vi "PB_VLIW_diagnostics4.vi"(3 "error in \n(no error)":errorcluster, 6 "VLIW Array In":T1(array[cluster]) {"OP Code" format="%.0x"; "Output Bits" format="%.0x"}) -> (0 "error out":errorcluster, 2 "Total Time":dbl=50.0 format="%.2p")   [LabVIEW 2012, in "SubVIs.lvlib"]
doc: "This vi obtains information about a \"VLIW Array\".\n\nIt's inputs are:\n1) the \"VLIW Array\"\n2) error in\nIt's outputs are:\n1) the total time for the sequence\n2) the total number of AO updates for each different AO/DO device specified in the HW Globals array\n3) error out. \n\n\nThe Jump, Return, and GoTo diagnostics are not supported, and attempting to determine diagnostics on an array that contains these commands will generate and error. If there is an error on the input, the diagnostics are not calculated.\n\nThis vi uses the globally defined variables in \"PB_defines\"."
uses:
  PB_defines.vi
  SubVIs.lvlib
  PulseBlaster.lvlib
panel:
  in  "Start loop time":dbl format="%.2p"
  in  "# of loops":u32
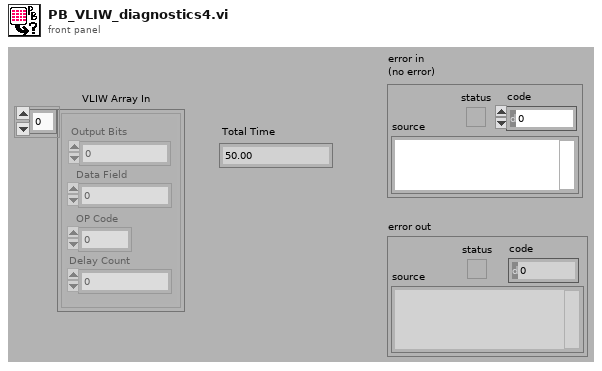
[diagram p1: front panel]
types:
  T1 = cluster{"Output Bits":u32, "Data Field":u32, "OP Code":u8, "Delay Count":u32}[]
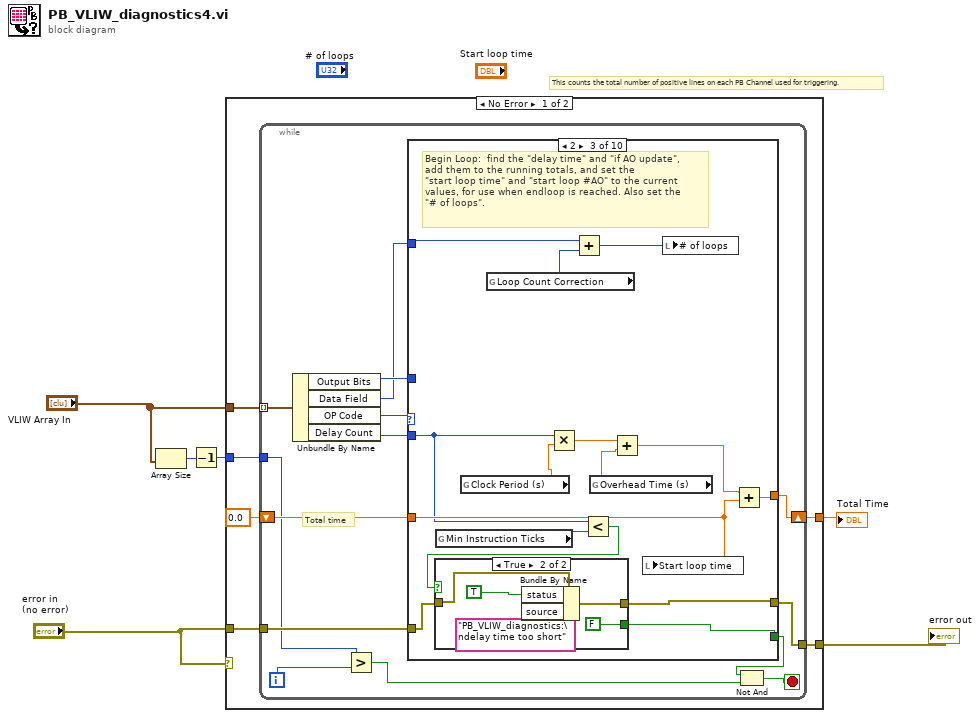
[diagram p0: block diagram]
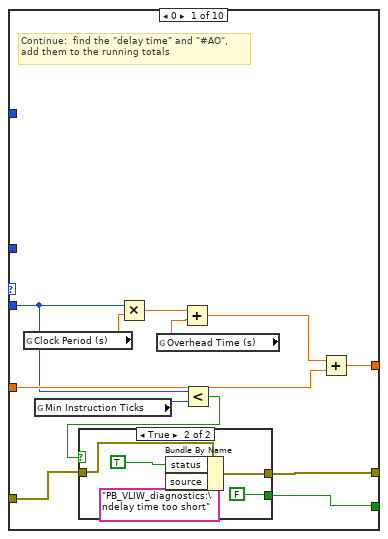
[diagram p2: hidden frame]
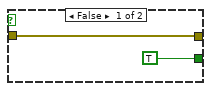
[diagram p3: hidden frame]
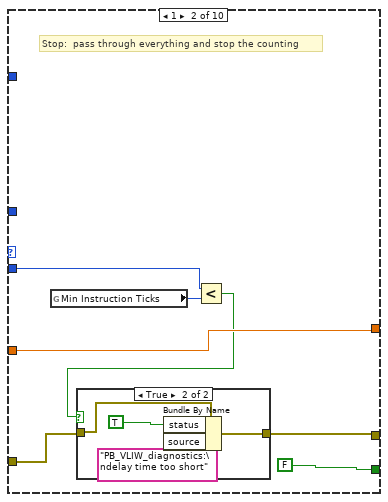
[diagram p4: hidden frame]
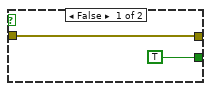
[diagram p6: hidden frame]
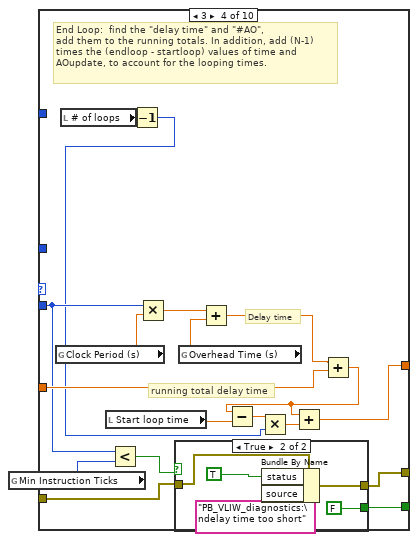
[diagram p7: hidden frame]
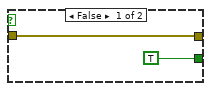
[diagram p8: hidden frame]
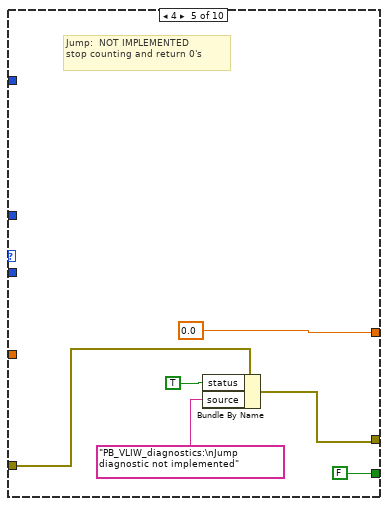
[diagram p9: hidden frame]
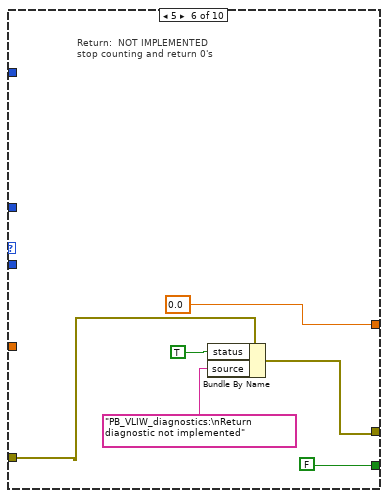
[diagram p10: hidden frame]
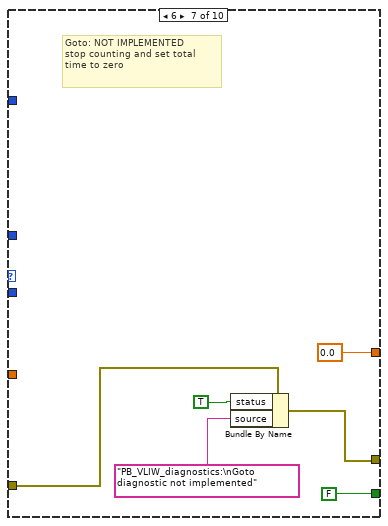
[diagram p11: hidden frame]
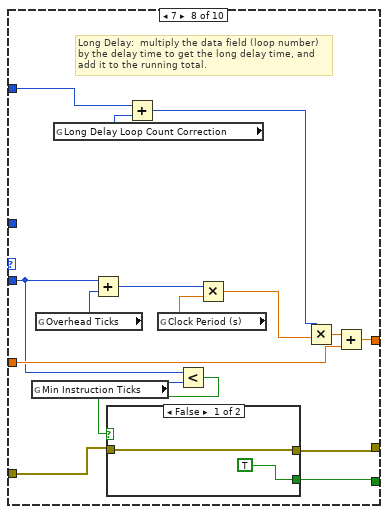
[diagram p12: hidden frame]
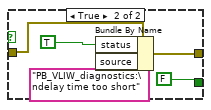
[diagram p13: hidden frame]
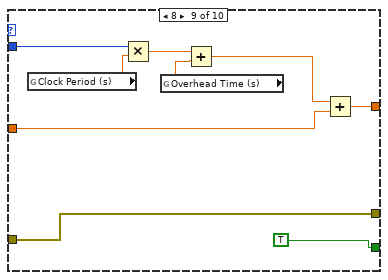
[diagram p14: hidden frame]
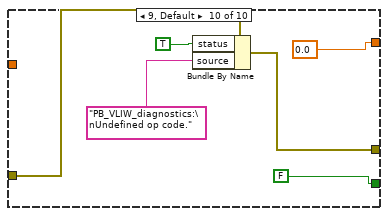
[diagram p15: hidden frame]
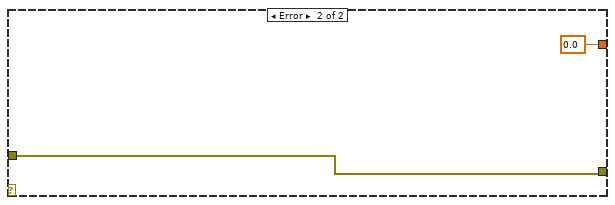
[diagram p16: hidden frame]
diagram:
  # "This counts the total number of positive lines on each PB Channel used for triggering."
  n1 = Array Size(array="VLIW Array In") -> (size(s)=w2:i32)
  n2 = Decrement(x=w2) -> (x-1=w1:i32)
  n3 = case shown="No Error" "error in \n(no error)" {
    tunnel: [w11 0.0] -> w6
    tunnel: "VLIW Array In" -> [w7 _]
    tunnel: "error in \n(no error)" -> [w10 w162]
    tunnel: [w9 w162] -> w5
    tunnel: w1 -> [w8 _]
    frame No Error {
      n4 = while {
        tunnel: w8 -> [w13]
        tunnel: [w18] -> w9
        tunnel: w10 -> [w19]
        shift-left: 0.0 -> [w25]
        shift-right: [w24] -> w11
        tunnel: w7 -> [w26] mode=indexing
        i -> [w14]
        stop <- w16 stop-if-true
        # "Total time"
        n5 = Unbundle By Name(w26) -> ("Output Bits"=w21:u32, "Data Field"=w20:u32, "OP Code"=w22:u8, "Delay Count"=w23:u32)
        n6 = Greater?(x=w13, y=w14) -> (0:w15:bool)
        n7 = case shown="2" w22 {
          tunnel: w23 -> [w31 w48 w61 w85 _ _ _ w126 w147 _]
          tunnel: w21 -> [_ _ _ _ _ _ _ _ _ _]
          tunnel: w25 -> [w34 w52 w62 w89 _ _ _ w127 w148 _]
          tunnel: [w35 w52 w68 w90 0.0 0.0 0.0 w133 w146 0.0] -> w24
          tunnel: [w27 FALSE w58 w82 FALSE FALSE FALSE w123 TRUE FALSE] -> w17
          tunnel: w20 -> [_ _ w66 _ _ _ _ w137 _ _]
          tunnel: w19 -> [w29 w51 w64 w87 w107 w113 w119 w128 w153 w157]
          tunnel: [w28 w50 w63 w83 w106 w112 w118 w129 w153 w156] -> w18
          frame 0 {
            # "Continue:  find the \"delay time\" and \"#AO\",\nadd them to the running totals"
            n8 = global read "PB_defines.vi" "Clock Period (s)"() -> (w37:dbl)
            n9 = global read "PB_defines.vi" "Min Instruction Ticks"() -> (w32:u8)
            n10 = Multiply(x=w31, y=w37) -> (x*y=w36:dbl)
            n11 = global read "PB_defines.vi" "Overhead Time (s)"() -> (w38:dbl)
            n12 = Add(x=w36, y=w38) -> (x+y=w33:dbl)
            n13 = Less?(x=w31, y=w32) -> (x < y?=w30:bool)
            n14 = case shown="True" w30 {
              tunnel: w29 -> [w40 w45]
              tunnel: [w40 w42] -> w28
              tunnel: [TRUE FALSE] -> w27
              frame False {
              }
              frame True {
                n15 = Bundle By Name(cluster=w45, "status"=TRUE, "source"="PB_VLIW_diagnostics:\ndelay time too short") -> (w42:errorcluster)
              }
            }
            n16 = Add(x=w33, y=w34) -> (x+y=w35:dbl)
          }
          frame 1 {
            # "Stop:  pass through everything and stop the counting"
            n17 = global read "PB_defines.vi" "Min Instruction Ticks"() -> (w49:u8)
            n18 = Less?(x=w48, y=w49) -> (x < y?=w47:bool)
            n19 = case shown="True" w47 {
              tunnel: w51 -> [w53 w57]
              tunnel: [w53 w54] -> w50
              frame False {
              }
              frame True {
                n20 = Bundle By Name(cluster=w57, "status"=TRUE, "source"="PB_VLIW_diagnostics:\ndelay time too short") -> (w54:errorcluster)
              }
            }
          }
          frame 2 {
            # "Begin Loop:  find the \"delay time\" and \"if AO update\",\nadd them to the running totals, and set the \n\"start loop time\" and \"start loop #AO\" to the current\nvalues, for use when endloop is reached. Also set the\n\"# of loops\"."
            n21 = global read "PB_defines.vi" "Min Instruction Ticks"() -> (w59:u8)
            n22 = global read "PB_defines.vi" "Clock Period (s)"() -> (w71:dbl)
            n23 = global read "PB_defines.vi" "Loop Count Correction"() -> (w67:u8)
            n24 = Multiply(x=w61, y=w71) -> (x*y=w70:dbl)
            n25 = Add(x=w66, y=w67) -> (x+y=w65:u32)
            n26 = Less?(x=w61, y=w59) -> (x < y?=w60:bool)
            n27 = case shown="True" w60 {
              tunnel: w64 -> [w74 w79]
              tunnel: [w74 w76] -> w63
              tunnel: [TRUE FALSE] -> w58
              frame False {
              }
              frame True {
                n28 = Bundle By Name(cluster=w79, "status"=TRUE, "source"="PB_VLIW_diagnostics:\ndelay time too short") -> (w76:errorcluster)
              }
            }
            n29 = global read "PB_defines.vi" "Overhead Time (s)"() -> (w72:dbl)
            n30 = Add(x=w70, y=w72) -> (x+y=w69:dbl)
            n31 = local write "Start loop time"(w62) -> ()
            n32 = local write "# of loops"(w65) -> ()
            n33 = Add(x=w69, y=w62) -> (x+y=w68:dbl)
          }
          frame 3 {
            # "running total delay time"
            # "Delay time"
            # "End Loop:  find the \"delay time\" and \"#AO\",\nadd them to the running totals. In addition, add (N-1)\ntimes the (endloop - startloop) values of time and\nAOupdate, to account for the looping times."
            n34 = global read "PB_defines.vi" "Min Instruction Ticks"() -> (w86:u8)
            n35 = global read "PB_defines.vi" "Clock Period (s)"() -> (w96:dbl)
            n36 = local read "# of loops"() -> (w80:u32)
            n37 = local read "Start loop time"() -> (w88:dbl)
            n38 = Less?(x=w85, y=w86) -> (x < y?=w84:bool)
            n39 = Decrement(x=w80) -> (x-1=w81:u32)
            n40 = Multiply(x=w85, y=w96) -> (x*y=w95:dbl)
            n41 = case shown="True" w84 {
              tunnel: w87 -> [w99 w104]
              tunnel: [w99 w101] -> w83
              tunnel: [TRUE FALSE] -> w82
              frame False {
              }
              frame True {
                n42 = Bundle By Name(cluster=w104, "status"=TRUE, "source"="PB_VLIW_diagnostics:\ndelay time too short") -> (w101:errorcluster)
              }
            }
            n43 = global read "PB_defines.vi" "Overhead Time (s)"() -> (w97:dbl)
            n44 = Add(x=w95, y=w97) -> (x+y=w94:dbl)
            n45 = Add(x=w94, y=w89) -> (x+y=w91:dbl)
            n46 = Subtract(x=w91, y=w88) -> (x-y=w93:dbl)
            n47 = Multiply(x=w93, y=w81) -> (x*y=w92:dbl)
            n48 = Add(x=w91, y=w92) -> (x+y=w90:dbl)
          }
          frame 4 {
            # "Jump:  NOT IMPLEMENTED\nstop counting and return 0's"
            n49 = Bundle By Name(cluster=w107, "status"=TRUE, "source"="PB_VLIW_diagnostics:\nJump diagnostic not implemented") -> (w106:errorcluster)
          }
          frame 5 {
            # "Return:  NOT IMPLEMENTED\nstop counting and return 0's"
            n50 = Bundle By Name(cluster=w113, "status"=TRUE, "source"="PB_VLIW_diagnostics:\nReturn diagnostic not implemented") -> (w112:errorcluster)
          }
          frame 6 {
            # "Goto: NOT IMPLEMENTED\nstop counting and set total\ntime to zero"
            n51 = Bundle By Name(cluster=w119, "status"=TRUE, "source"="PB_VLIW_diagnostics:\nGoto diagnostic not implemented") -> (w118:errorcluster)
          }
          frame 7 {
            # "Long Delay:  multiply the data field (loop number)\nby the delay time to get the long delay time, and\nadd it to the running total."
            n52 = global read "PB_defines.vi" "Min Instruction Ticks"() -> (w124:u8)
            n53 = global read "PB_defines.vi" "Overhead Ticks"() -> (w138:u8)
            n54 = global read "PB_defines.vi" "Long Delay Loop Count Correction"() -> (w136:u8)
            n55 = Add(x=w126, y=w138) -> (x+y=w135:u32)
            n56 = Add(x=w137, y=w136) -> (x+y=w130:u32)
            n57 = global read "PB_defines.vi" "Clock Period (s)"() -> (w134:dbl)
            n58 = Less?(x=w126, y=w124) -> (x < y?=w125:bool)
            n59 = case shown="False" w125 {
              tunnel: w128 -> [w140 w145]
              tunnel: [w140 w142] -> w129
              tunnel: [TRUE FALSE] -> w123
              frame False {
              }
              frame True {
                n60 = Bundle By Name(cluster=w145, "status"=TRUE, "source"="PB_VLIW_diagnostics:\ndelay time too short") -> (w142:errorcluster)
              }
            }
            n61 = Multiply(x=w135, y=w134) -> (x*y=w131:dbl)
            n62 = Multiply(x=w130, y=w131) -> (x*y=w132:dbl)
            n63 = Add(x=w132, y=w127) -> (x+y=w133:dbl)
          }
          frame 8 {
            n64 = global read "PB_defines.vi" "Clock Period (s)"() -> (w151:dbl)
            n65 = Multiply(x=w147, y=w151) -> (x*y=w150:dbl)
            n66 = global read "PB_defines.vi" "Overhead Time (s)"() -> (w152:dbl)
            n67 = Add(x=w150, y=w152) -> (x+y=w149:dbl)
            n68 = Add(x=w149, y=w148) -> (x+y=w146:dbl)
          }
          frame 9, Default {
            n69 = Bundle By Name(cluster=w157, "status"=TRUE, "source"="PB_VLIW_diagnostics:\nUndefined op code.") -> (w156:errorcluster)
          }
        }
        n70 = Not And(1:w15, 2:w17) -> (0:w16:bool)
      }
    }
    frame Error {
    }
  }
  "error out" <- w5
  "Total Time" <- w6
